vi "Check Mode Delay Update.vi"(7 "TreeControl in":refnum<vi>, 8 "Analog Changed":bool=TRUE, 9 "New Num":i32, 10 "Settings In in":T1, 11 "Tree Data in":cluster{"Tag":string[], "Settings":T3[]} {"Settings"."Data Type" items=["Tree Parent"=-1, "Numeric"=0, "String"=1, "Boolean"=2, "Enum"=3]}) -> (3 "Tree Data out":cluster{"Tag":string[], "Settings":T3[]} {"Settings"."Data Type" items=["Tree Parent"=-1, "Numeric"=0, "String"=1, "Boolean"=2, "Enum"=3]})   [LabVIEW 2024, in "Sequencer with Output Values.lvlib" / "Sequencer with Output Values.lvclass"]
uses:
  Sequencer with Output Values.lvclass
  Tree Item Settings.ctl
  Data Type.ctl
  Params.ctl
  Step Settings.ctl
  Global Tree Data.vi
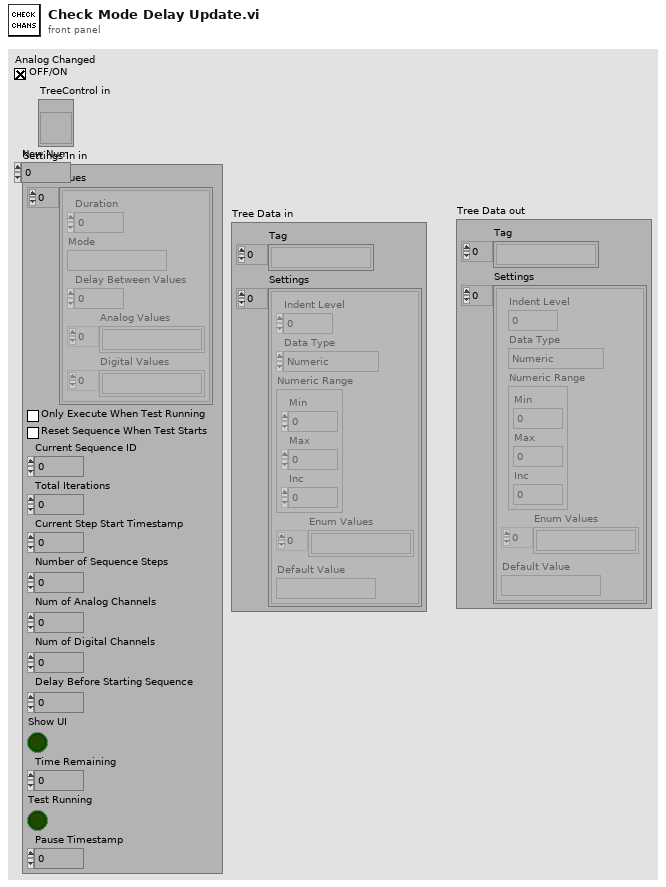
[diagram p1: front panel]
types:
  T1 = typedef "Sequencer with Output Values.lvlib/Sequencer with Output Values.lvclass/Params.ctl" = cluster{"Step Values":T2[], "Only Execute When Test Running":bool, "Reset Sequence When Test Starts":bool, "Current Sequence ID":u32, "Total Iterations":u32, "Current Step Start Timestamp":dbl, "Number of Sequence Steps":i32, "Num of Analog Channels":i32, "Num of Digital Channels":i32, "Delay Before Starting Sequence":dbl, "Show UI":bool, "Time Remaining":dbl, "Test Running":bool, "Pause Timestamp":dbl}
  T2 = typedef "Sequencer with Output Values.lvlib/Sequencer with Output Values.lvclass/Step Settings.ctl" = cluster{"Duration":dbl, "Mode":string, "Delay Between Values":dbl, "Analog Values":string[], "Digital Values":string[]}
  T3 = typedef "Sequencer with Output Values.lvlib/Sequencer with Output Values.lvclass/Tree Item Settings.ctl" = cluster{"Indent Level":i32, "Data Type":T4, "Numeric Range":cluster{"Min":dbl, "Max":dbl, "Inc":dbl}, "Enum Values":string[], "Default Value":string}
  T4 = typedef "Sequencer with Output Values.lvlib/Sequencer with Output Values.lvclass/Data Type.ctl" = i16
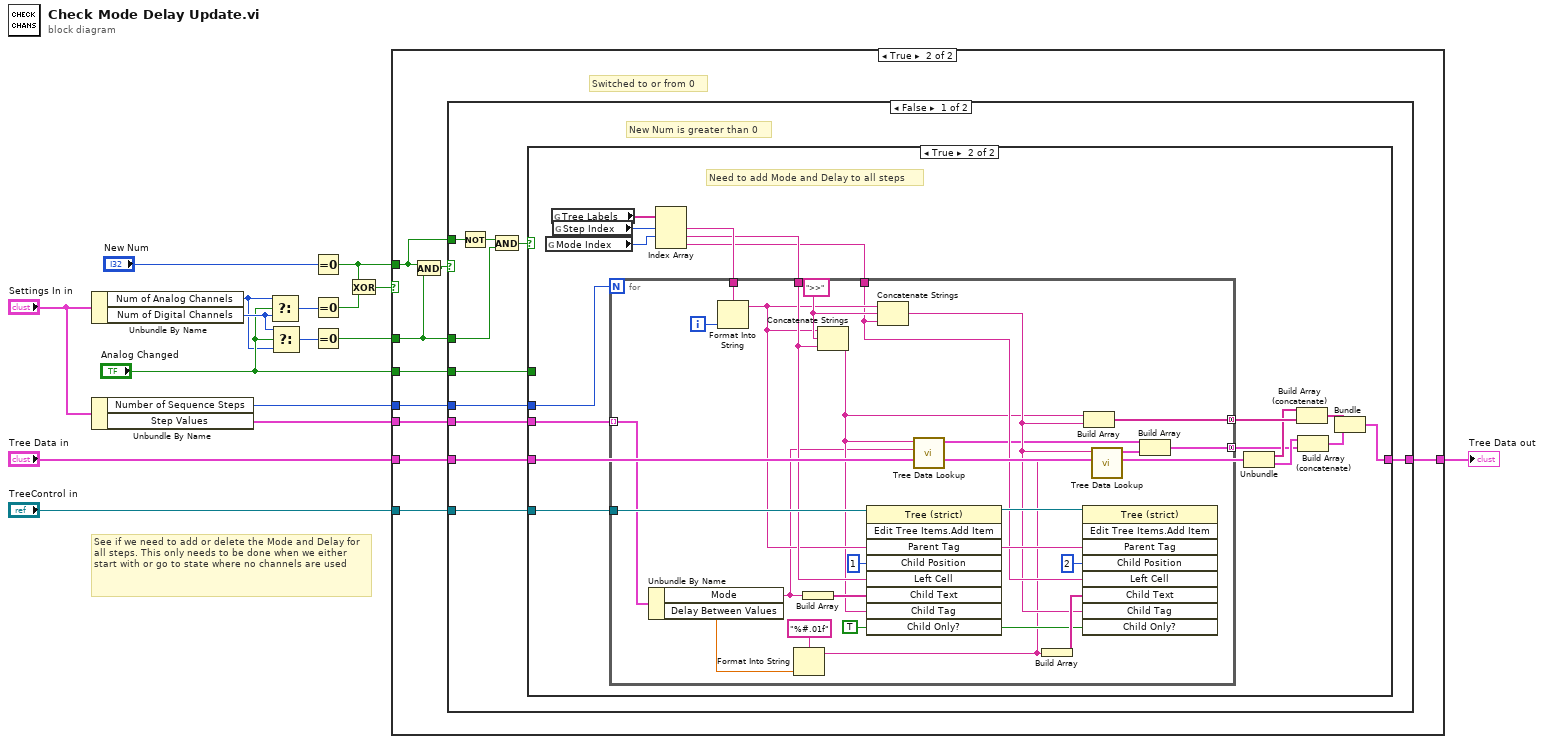
[diagram p0: block diagram]
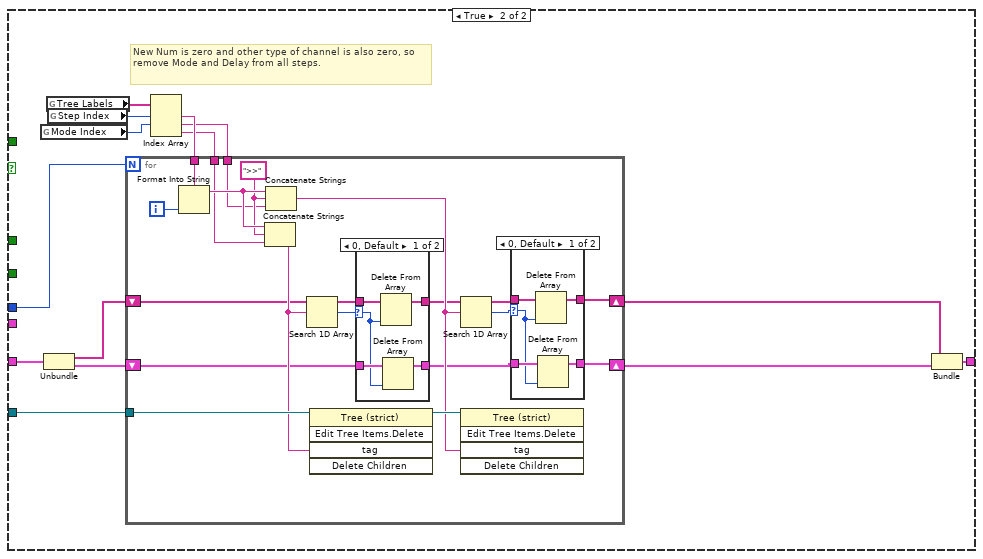
[diagram p4: hidden frame]
diagram:
  # "See if we need to add or delete the Mode and Delay for all steps. This only needs to be done when we either start with or go to state where no channels are used"
  n1 = Unbundle By Name("Settings In in") -> ("Num of Analog Channels"=w1:i32, "Num of Digital Channels"=w11:i32)
  n2 = Unbundle By Name("Settings In in") -> ("Number of Sequence Steps"=w5:i32, "Step Values"=w2:T2[])
  n3 = Select(t=w1, s="Analog Changed", f=w11) -> (s? t:f=w15:i32)
  n4 = Select(t=w11, s="Analog Changed", f=w1) -> (s? t:f=w10:i32)
  n5 = Equal To 0?(x="New Num") -> (x = 0?=w12:bool)
  n6 = Equal To 0?(x=w15) -> (x = 0?=w14:bool)
  n7 = Equal To 0?(x=w10) -> (x = 0?=w9:bool)
  n8 = Exclusive Or(1:w14, 2:w12) -> (0:w13:bool)
  n9 = case shown="True" w13 {
    tunnel: w12 -> [_ w21]
    tunnel: w9 -> [_ w20]
    tunnel: "TreeControl in" -> [_ w25]
    tunnel: "Tree Data in" -> [w17 w24]
    tunnel: w5 -> [_ w23]
    tunnel: [w17 w22] -> w4
    tunnel: "Analog Changed" -> [_ w19]
    tunnel: w2 -> [_ w18]
    frame False {
      # "Change didn't affect if we should or should not display Mode and Delay"
    }
    frame True {
      # "Switched to or from 0"
      n10 = And(x=w21, y=w20) -> (x .and. y?=w26:bool)
      n11 = case shown="False" w26 {
        tunnel: w25 -> [w29 w87]
        tunnel: w24 -> [w32 w84]
        tunnel: w23 -> [w28 w92]
        tunnel: [w31 w79] -> w22
        tunnel: w21 -> [w36 _]
        tunnel: w20 -> [w34 _]
        tunnel: w19 -> [w30 _]
        tunnel: w18 -> [w27 _]
        frame False {
          # "New Num is greater than 0"
          n12 = Not(x=w36) -> (.not. x?=w35:bool)
          n13 = And(x=w35, y=w34) -> (x .and. y?=w33:bool)
          n14 = case shown="True" w33 {
            tunnel: w32 -> [w37 w45]
            tunnel: [w37 w38] -> w31
            tunnel: w30 -> [_ _]
            tunnel: w29 -> [_ w54]
            tunnel: w28 -> [_ w50]
            tunnel: w27 -> [_ w47]
            frame False {
            }
            frame True {
              # "Need to add Mode and Delay to all steps"
              n15 = global read "Global Tree Data.vi" "Mode Index"() -> (w51:i32)
              n16 = global read "Global Tree Data.vi" "Tree Labels"() -> (w53:string[])
              n17 = global read "Global Tree Data.vi" "Step Index"() -> (w52:i32)
              n18 = Index Array(array=w53, index #1=w52, index #2=w51) -> (element #1=w49:string, element #2=w48:string, element #3=w46:string)  [unwired: 1 in]
              n19 = for {
                N: w50 -> [_]
                tunnel: w54 -> [w78]
                tunnel: w49 -> [w77]
                tunnel: w48 -> [w75]
                tunnel: w47 -> [w73] mode=indexing
                tunnel: w46 -> [w67]
                tunnel: [w61] -> w44 mode=concatenating
                tunnel: [w55] -> w41 mode=concatenating
                i -> [w76]
                w63 = TRUE ("Child Only?")
                w70 = ">>" ("string")
                n20 = Unbundle By Name(w73) -> ("Mode"=w57:string, "Delay Between Values"=w66:dbl)
                n21 = Format Into String(format string=w77, w76) -> (resulting string=w69:string)  [unwired: 2 in, 1 out]
                n22 = Format Into String(format string="%#.01f", w66) -> (resulting string=w60:string)  [unwired: 2 in, 1 out]
                n23 = Build Array(w57) -> (w72:string[])
                n24 = Concatenate Strings(w69, w70, w75) -> (w58:string)
                n25 = invoke class="Tree (strict)" method="Edit Tree Items.Add Item"(reference=w78, "Parent Tag"=w69, "Child Position"=1, "Left Cell"=w75, "Child Text"=w72, "Child Tag"=w58, "Child Only?"=w63) -> (reference out=w71:refnum<vi>)  [unwired: 2 in, 8 out]
                n26 = Concatenate Strings(w69, w70, w67) -> (w62:string)
                n27 = call "Tree Data Lookup.vi"("Value"=w57, "Key"=w58) -> ("Tree Data"=w56:T3)  [unwired: 9 in]
                n28 = Build Array(w60) -> (w64:string[])
                n29 = invoke class="Tree (strict)" method="Edit Tree Items.Add Item"(reference=w71, "Parent Tag"=w69, "Child Position"=2, "Left Cell"=w67, "Child Text"=w64, "Child Tag"=w62, "Child Only?"=w63) -> ()  [unwired: 2 in, 9 out]
                n30 = Build Array(w58, w62) -> (w61:string[])
                n31 = call "Tree Data Lookup.vi"("Value"=w60, "Key"=w62) -> ("Tree Data"=w59:T3)  [unwired: 9 in]
                n32 = Build Array(w56, w59) -> (w55:T3[])
              }
              n33 = Unbundle(w45) -> ("Tag"=w43:string[], "Settings"=w42:T3[])
              n34 = Build Array (concatenate)(w43, w44) -> (w40:string[])
              n35 = Build Array (concatenate)(w42, w41) -> (w39:T3[])
              n36 = Bundle(w40, w39) -> (w38:cluster{string[], T3[]})  [unwired: 1 in]
            }
          }
        }
        frame True {
          # "New Num is zero and other type of channel is also zero, so remove Mode and Delay from all steps."
          n37 = global read "Global Tree Data.vi" "Mode Index"() -> (w89:i32)
          n38 = Unbundle(w84) -> ("Tag"=w83:string[], "Settings"=w82:T3[])
          n39 = global read "Global Tree Data.vi" "Tree Labels"() -> (w91:string[])
          n40 = global read "Global Tree Data.vi" "Step Index"() -> (w90:i32)
          n41 = Index Array(array=w91, index #1=w90, index #2=w89) -> (element #1=w88:string, element #2=w86:string, element #3=w85:string)  [unwired: 1 in]
          n42 = for {
            N: w92 -> [_]
            tunnel: w88 -> [w110]
            tunnel: w87 -> [w108]
            tunnel: w86 -> [w105]
            tunnel: w85 -> [w104]
            shift-right: [w94] -> w80
            shift-left: w83 -> [w99]
            shift-right: [w93] -> w81
            shift-left: w82 -> [w100]
            i -> [w109]
            w106 = ">>" ("string")
            n43 = Format Into String(format string=w110, w109) -> (resulting string=w107:string)  [unwired: 2 in, 1 out]
            n44 = Concatenate Strings(w107, w106, w104) -> (w102:string)
            n45 = Concatenate Strings(w107, w106, w105) -> (w98:string)
            n46 = Search 1D Array(1D array=w99, element=w102) -> (index of element=w101:i32)  [unwired: 1 in]
            n47 = invoke class="Tree (strict)" method="Edit Tree Items.Delete"(reference=w108, "tag"=w102) -> (reference out=w103:refnum<vi>)  [unwired: 3 in, 4 out]
            n48 = case shown="0, Default" w101 {
              selector: w101 -> [w120 _]
              tunnel: w100 -> [w121 w123]
              tunnel: w99 -> [w122 w124]
              tunnel: [w119 w124] -> w96
              tunnel: [w118 w123] -> w95
              frame 0, Default {
                n49 = Delete From Array(array=w122, index=w120) -> (array with subset deleted=w119:string[])  [unwired: 1 in, 1 out]
                n50 = Delete From Array(array=w121, index=w120) -> (array with subset deleted=w118:T3[])  [unwired: 1 in, 1 out]
              }
              frame -1 {
              }
            }
            n51 = Search 1D Array(1D array=w96, element=w98) -> (index of element=w97:i32)  [unwired: 1 in]
            n52 = invoke class="Tree (strict)" method="Edit Tree Items.Delete"(reference=w103, "tag"=w98) -> ()  [unwired: 3 in, 5 out]
            n53 = case shown="0, Default" w97 {
              selector: w97 -> [w113 _]
              tunnel: w95 -> [w114 w116]
              tunnel: w96 -> [w115 w117]
              tunnel: [w112 w117] -> w94
              tunnel: [w111 w116] -> w93
              frame 0, Default {
                n54 = Delete From Array(array=w115, index=w113) -> (array with subset deleted=w112:string[])  [unwired: 1 in, 1 out]
                n55 = Delete From Array(array=w114, index=w113) -> (array with subset deleted=w111:T3[])  [unwired: 1 in, 1 out]
              }
              frame -1 {
              }
            }
          }
          n56 = Bundle("Tag"=w80, "Settings"=w81) -> (w79:cluster{"Tag":string[], "Settings":T3[]})  [unwired: 1 in]
        }
      }
    }
  }
  "Tree Data out" <- w4
